vi "linear_height.vi"() -> ()   [LabVIEW 2015]
panel:
  in  "Open DB":bool
  # "Note preliminari alla misura:\n\n1) Affiancare alla barra da misurare un metro estensibile per facilitare\n    la misura\n2) Inserire una chiavetta USB nello strumento PRIMA di accenderlo\n\nImpostazione del programma di misura:\n\n1) Premere il pulsante \"RUN\"\n2) Selezionare il programma \"frame\"\n3) Confermare la richiesta di \"Esecuzione passo\"\n4) Impostare il numero di misure (NOTA: per una camera completa sono \n    necessarie 86 misure)\n5) Effetture tre misure ogni 10 cm, una sulla parte centrale e sui due bordi\n\nProcedimento:\n\n1) Calibrare il LH impostando lo zero.\n2) Effettuare tre misure ogni 10 cm sulla faccia superiore (Figura 1 e 2) e\n    analogamente sulla faccia inferiore\n3) Effettuare una misura ogni 10 cm sul bordo sinistro e destro"
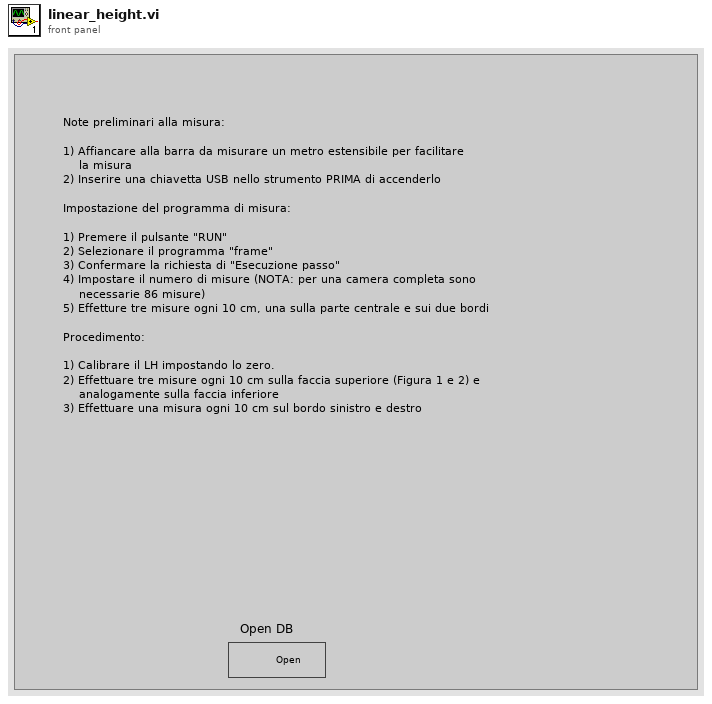
[diagram p1: front panel]
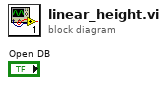
[diagram p0: block diagram]
diagram:
